vi "Setup.vi"(8 "error in (no error)":errorcluster, 11 "Process Test In":refnum<class "Process Dev Test.lvclass">) -> (0 "error out":errorcluster, 3 "Process Test Out":refnum<class "Process Dev Test.lvclass">)   [LabVIEW 2020, in "Process Dev Test.lvclass"]
uses:
  Process Dev Test.lvclass
  C:/Git/astemes-triarc-framework/source/Framework Test/Base Class Test/Base Test.lvclass
  source/Framework/Process/Process.lvclass
  C:/Git/astemes-triarc-framework/source/Framework/Base/Base.lvclass
  source/Framework Test Suite/Base Class Test/Base Test.lvclass/Base Test.ctl
  Process Dev Test.lvclass/Process Dev Test.ctl
  source/Framework Test Suite/Base Class Test/Base Test.lvclass
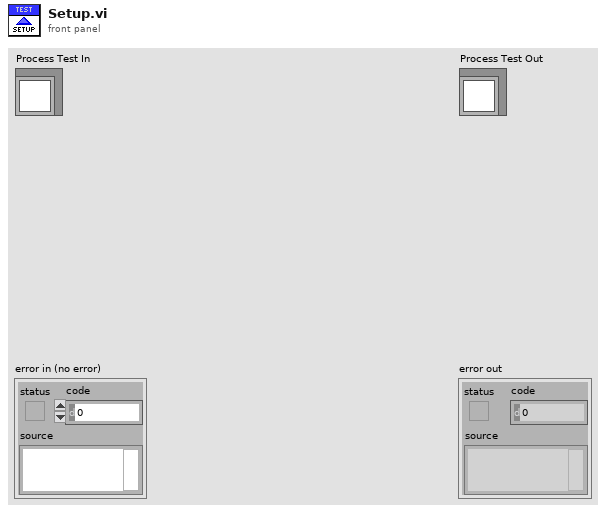
[diagram p1: front panel]
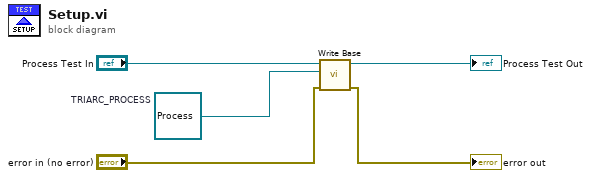
[diagram p0: block diagram]
diagram:
  w3 = refnum<class "Process.lvclass"> refnum  # TRIARC_PROCESS
  n1 = call "Write Base.vi"("error in (no error)"="error in (no error)", "Base"=w3, "Base Class Test In"="Process Test In") -> ("error out"=→"error out":errorcluster, "Base Class Test Out"=→"Process Test Out":refnum<class "Process Dev Test.lvclass">)  [unwired: 7 in]
